vi "DigitizerConfigGain.vi"(8 "error in (no error)":errorcluster, 10 "FLImDAQ":T1={"Digitizer 1"="PXI1Slot3", "Digitizer 2"="PXI1Slot4", "Channel"=enum."Channel 0", "trigger source"="VAL_EXTERNAL", "trigger level"=0.5, "trigger delay"=1.35e-07, "min sample rate"=12500000000.0, "min record length"=2500, "vertical range"=1.0, "vertical offset"=-0.25, "Waveform to Avg"=2000} caption="FLIm DAQ Configuration" {"trigger delay" format="%^#.4e"; "trigger level" min=0.0 max=3.5 step=0.5 format="%.2f"; "vertical offset" format="%.4f"; "vertical range" format="%.2f"; "min sample rate" format="%#.2p"}, 11 "IVI Refnum in":refnum<k15>) -> (0 "error out":errorcluster, 3 "IVI Refnum out":refnum<k15>)   [LabVIEW 2020]
uses:
  FLImDAQ.ctl
  <instrlib>/niScope/Controls/niScope trigger source.ctl
  <instrlib>/niScope/Controls/niScope vertical coupling.ctl
  <instrlib>/niScope/Configure/Trigger/niScope Configure Trigger Immediate.vi
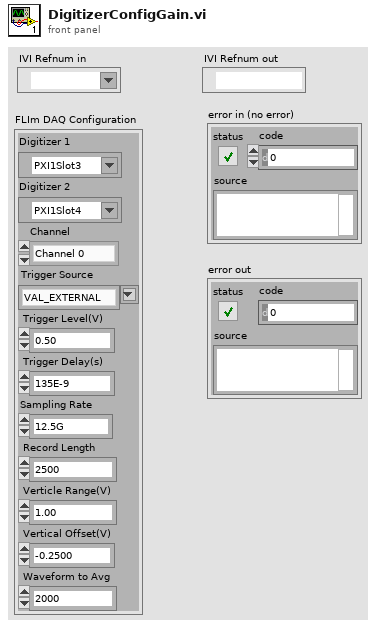
[diagram p1: front panel]
types:
  T1 = typedef "FLImDAQ.ctl" = cluster{"Digitizer 1":refnum<k15>, "Digitizer 2":refnum<k15>, "Channel":enum16{"Channel 0", "Channel 1", "Channel 0&1"}, "trigger source":T2, "trigger level":dbl, "trigger delay":dbl, "min sample rate":dbl, "min record length":i32, "vertical range":dbl, "vertical offset":dbl, "Waveform to Avg":i16}
  T2 = typedef "niScope trigger source.ctl" = string
  T3 = typedef "niScope vertical coupling.ctl" = i32
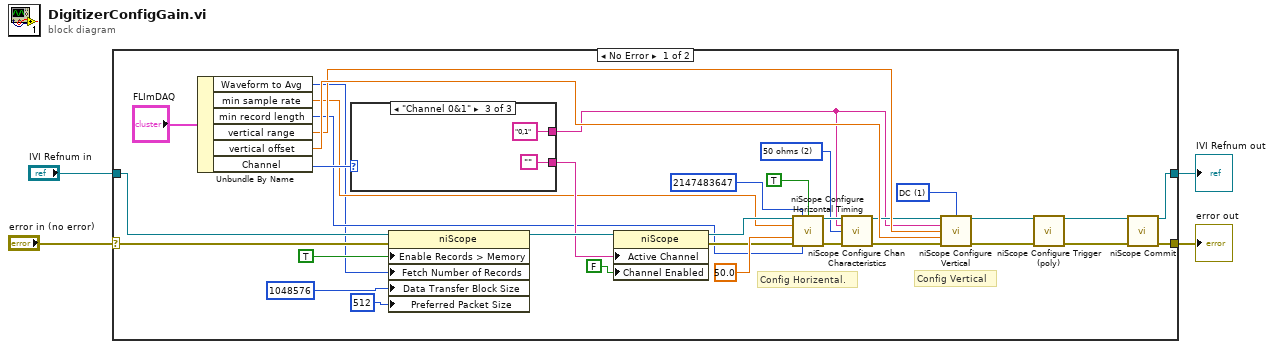
[diagram p0: block diagram]
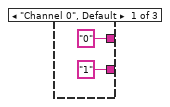
[diagram p2: hidden frame]
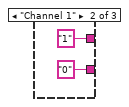
[diagram p3: hidden frame]
diagram:
  n1 = case shown="No Error" "error in (no error)" {
    selector: "error in (no error)" -> [w19 w45]
    tunnel: [w37 w44] -> w4
    tunnel: [w31 w45] -> w3
    tunnel: "IVI Refnum in" -> [w21 w44]
    frame No Error {
      w23 = u32 2 items=["1 mega ohm"=0, "50 ohms"=2] ("input impedance")
      w36 = T3 1 items=["AC", "DC", "Ground"] ("vertical coupling")
      # "Config Vertical"
      # "Config Horizental."
      n2 = Unbundle By Name("FLImDAQ") -> ("Waveform to Avg"=w5:i16, "min sample rate"=w7:dbl, "min record length"=w6:i32, "vertical range"=w32:dbl, "vertical offset"=w35:dbl, "Channel"=w29:enum16{"Channel 0", "Channel 1", "Channel 0&1"})
      n3 = case shown="\"Channel 0&1\"" w29 {
        tunnel: ["0" ("channels") "1" ("channels") "0,1" ("channels")] -> w15
        tunnel: ["1" ("channels") "0" ("channels") ""] -> w13
        frame "Channel 0", Default {
        }
        frame "Channel 1" {
        }
        frame "Channel 0&1" {
        }
      }
      n4 = property class="niScope"(reference=w21, error in=w19, "Enable Records > Memory"=TRUE ("Horizontal:Enable Records > Memory"), "Fetch Number of Records"=w5, "Data Transfer Block Size"=1048576 ("Fetch:Data Transfer Block Size"), "Preferred Packet Size"=512 ("Fetch:Advanced:Preferred Packet Size")) -> (reference out=w14:refnum<k15>)  [unwired: 1 out]
      n5 = property class="niScope"(reference=w14, "Active Channel"=w13, "Channel Enabled"=FALSE ("Vertical:Channel Enabled")) -> (reference out=w11:refnum<k15>, error out=w10:errorcluster)  [unwired: 1 in]
      n6 = call <instrlib>:"niScope Configure Horizontal Timing.vi"("instrument handle"=w11, "number of records"=2147483647, "enforce realtime"=TRUE, "min sample rate"=w7, "reference position"=50.0, "error in"=w10, "min record length"=w6) -> ("instrument handle out"=w27:refnum<k15>, "error out"=w25:errorcluster)  [unwired: 7 in]
      n7 = call <instrlib>:"niScope Configure Chan Characteristics.vi"("instrument handle"=w27, "channels"=w15, "input impedance"=w23, "error in"=w25) -> ("instrument handle out"=w26:refnum<k15>, "error out"=w24:errorcluster)  [unwired: 10 in]
      n8 = call <instrlib>:"niScope Configure Vertical.vi"("instrument handle"=w26, "vertical coupling"=w36, "channels"=w15, "vertical range"=w32, "vertical offset"=w35, "error in"=w24) -> ("instrument handle out"=w34:refnum<k15>, "error out"=w33:errorcluster)  [unwired: 8 in]
      n9 = call-poly <instrlib>:"niScope Configure Trigger (poly).vi"("instrument handle"=w34, "error in"=w33) -> ("instrument handle out"=w9:refnum<k15>, "error out"=w8:errorcluster)  [unwired: 12 in]
      n10 = call <instrlib>:"niScope Commit.vi"("instrument handle"=w9, "error in"=w8) -> ("instrument handle out"=w37:refnum<k15>, "error out"=w31:errorcluster)  [unwired: 12 in]
    }
    frame Error {
    }
  }
  "IVI Refnum out" <- w4
  "error out" <- w3
